vi "Check Aurora Status.vi"(8 "error in":errorcluster, 11 "session In":T2) -> (0 "error out":errorcluster, 1 "USRP Aurora Status":T3(array[cluster]), 2 "USRP Aurora Errors":cluster{"crc_errors":i32, "overflows":i32}[](array[cluster]), 3 "session out":T1)   [LabVIEW 2023]
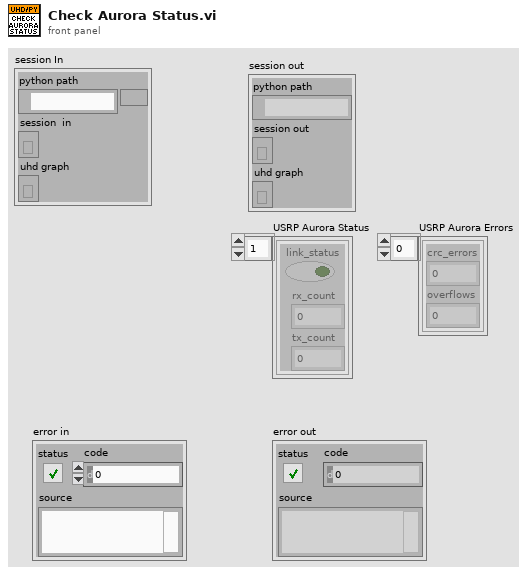
[diagram p1: front panel]
types:
  T1 = cluster{"python path":path, "session out":refnum<k35>, "uhd graph":refnum<k38>}
  T2 = cluster{"python path":path, "session  in":refnum<k35>, "uhd graph":refnum<k38>}
  T3 = cluster{"link_status":bool, "rx_count":i32, "tx_count":i32}[]
  T4 = cluster{"link status":bool, "rx_count":i32, "tx_count":i32}[]
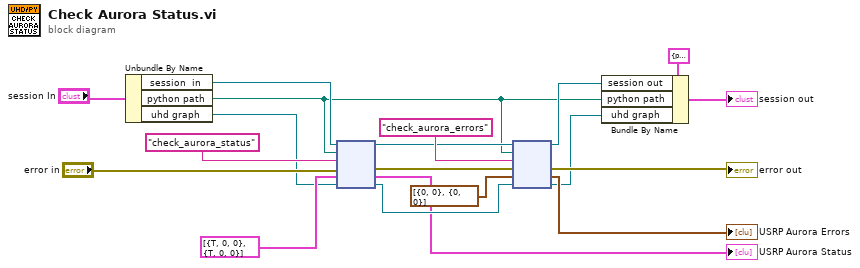
[diagram p0: block diagram]
diagram:
  n1 = Unbundle By Name("session In") -> ("session  in"=w8:refnum<k35>, "python path"=w4:path, "uhd graph"=w7:refnum<k38>)
  n2 = node(w8, w4, "check_aurora_status" ("function name"), "error in", T4 [{"link status"=TRUE, "rx_count"=0, "tx_count"=0}, {"link status"=TRUE, "rx_count"=0, "tx_count"=0}], w7) -> (w14:refnum<k35>, w16:errorcluster, →"USRP Aurora Status":T4, w10:refnum<k38>)  [unwired: 2 out]
  n3 = node(w14, w4, "check_aurora_errors" ("function name"), w16, cluster{"crc_errors":i32, "overflows":i32}[] [{"crc_errors"=0, "overflows"=0}, {"crc_errors"=0, "overflows"=0}], w10) -> (w5:refnum<k35>, →"error out":errorcluster, →"USRP Aurora Errors":cluster{"crc_errors":i32, "overflows":i32}[], w3:refnum<k38>)  [unwired: 2 out]
  n4 = Bundle By Name(cluster=T1 {"python path"=path "", "session out"=refnum, "uhd graph"=refnum}, "session out"=w5, "python path"=w4, "uhd graph"=w3) -> (→"session out":T1)
